vi "VGS Volume.vi"() -> ()   [LabVIEW 2022 SP3, in "LV_VGS.lvlib"]
uses:
  LV_VGS.lvlib
  typedefs/3D Size (I32).ctl
  RemoteControlClient/VGS_RemoteControlClient.lvclass
  Project/VGS_Project.lvclass
  VolumeDescriptor+File/VGS_VolumeDescriptor+File.lvclass
  VolumeDescriptor/VGS_VolumeDescriptor.lvclass
  ManufacturerInfo/VGS_ManufacturerInfo.lvclass
  ComponentInfo/VGS_ComponentInfo.lvclass
panel:
  out "Save Time, ms":u32
  # "Original Volume Example rewritten in LabVIEW"
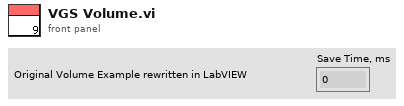
[diagram p1: front panel]
types:
  T1 = typedef "LV_VGS.lvlib/3D Size (I32).ctl" = cluster{"X":i32, "Y":i32, "Z":i32}
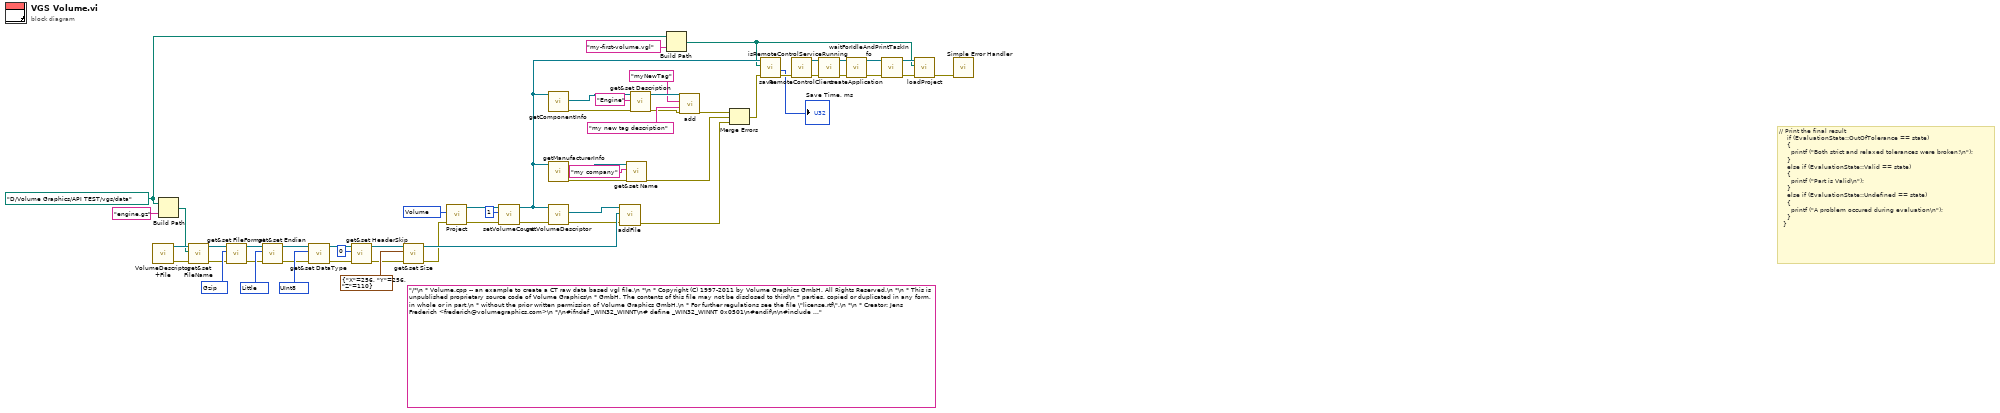
[diagram p0: block diagram]
diagram:
  w1 = 1448153088 items=["Volume"=1448153088, "Reconstruction"=1448153089] ("type")
  w46 = 1448157376 items=["UInt8"=1448157376, "Int8"=1448157377, "UInt16"=1448157378, "Int16"=1448157379, "UInt32"=1448157380, "Int32"=1448157381, "Float"=1448157382, "Rgb8"=1448157383] ("DataType")
  w49 = 1448157440 items=["Little"=1448157440, "Big"=1448157441] ("Endian")
  w52 = 1448157313 items=["Raw"=1448157312, "Gzip"=1448157313, "Tiff"=1448157314, "Jpeg"=1448157315, "Bmp"=1448157316, "Bir"=1448157317, "Toshiba"=1448157318, "Shimadzu"=1448157319, "Pnm"=1448157320, "Jpeg2"=1448157321, "Yxlon"=1448157322, "Hdf"=1448157323, "Dicom"=1448157324, "Imtec"=1448157325, "Aracor"=1448157326, "Fhg"=1448157327] ("FileFormat")
  w3 = path "D:/Volume Graphics/API TEST/vgs/data" ("replacementPattern")
  (unwired) "/*\n * Volume.cpp -- an example to create a CT raw data based vgl file.\n *\n * Copyright (C) 1997-2011 by Volume Graphics GmbH. All Rights Reserved.\n *\n * This is unpublished proprietary source code of Volume Graphics\n * GmbH. The contents of this file may not be disclosed to third\n * parties, copied or duplicated in any form, in whole or in part,\n * without the prior written permission of Volume Graphics GmbH.\n * For further regulations see the file \"license.rtf\".\n *\n * Creator: Jens Frederich <frederich@volumegraphics.com>\n */\n#ifndef _WIN32_WINNT\n# define _WIN32_WINNT 0x0501\n#endif\n\n#include <tchar.h>\n\n#include <vgs.project/project.h>\n\nusing namespace vgs::project;\nusing namespace vgs::project::volume;\n\nint _tmain (int argc, _TCHAR* argv[])\n{\n  Project* p = new Project (Project::Type::Volume);\n  assert (p != NULL);\n\n  // add single raw block file\n  {\n    VolumeDescriptor::File data;\n\n    data.setFileName   (\"D:/Volume Graphics/API TEST/vgs/data/engine.gz\");\n    data.setFileFormat (volume::FileFormat::Gzip);\n    data.setEndian     (volume::Endian::Little);\n    data.setDataType   (DataType::UInt8);\n    data.setHeaderSkip (0);\n    data.setSize       (Vector3<int> (256, 256, 110));\n    \n    p->setVolumeCount (1);\n    VolumeDescriptor* vd = p->getVolumeDescriptor (0);\n    assert (vd != NULL);\n\n    vd->addFile (data);\n  }\n\n  // add some meta data\n  {\n    ManufacturerInfo* mi = p->getManufacturerInfo ();\n    mi->setName (\"My company\");\n\n    ComponentInfo* ci = p->getComponentInfo ();\n    ci->setDescription (\"Engine\");\n\n    // add user defined tag\n    ci->add (\"myNewTag\", \"my new tag description\");\n\n    // add logo and preview\n    //p->setLogo    (\"c:/data/logo.png\");\n    //p->setPreview (\"c:/data/scene_preview.png\");\n  }\n\n  // create VG project\n  {\n    bool ok = true;\n\n    ok = p->save (std::string (\"D:/Volume Graphics/API TEST/vgs/data/my-first-volume1.vgl\"));\n    if (true != ok)\n    {\n      Error::ErrorCode err = Error::getLastError ();\n\t  printf(\"something is wrong, error code = %d\", err);\n      __debugbreak ();\n    }\n  }\n\n  // cleanup\n  if (p != NULL)\n  {\n    delete p;\n  }\n\n  return 0;\n}\n\n"
  # "// Print the final result\n    if (EvaluationState::OutOfTolerance == state)\n    {\n      printf (\"Both strict and relaxed tolerances were broken!\\n\");\n    }\n    else if (EvaluationState::Valid == state)\n    {\n      printf (\"Part is Valid\\n\");\n    }\n    else if (EvaluationState::Undefined == state)\n    {\n      printf (\"A problem occured during evaluation\\n\");\n    }\n  }"
  n1 = call "VolumeDescriptor+File.vi"() -> ("error out"=w54:errorcluster, "VGS_VolumeDescriptor+File out"=w57:refnum<class "VGS_VolumeDescriptor+File.lvclass">)  [unwired: 10 in]
  n2 = Build Path(base path=w3, name or relative path="engine.gz") -> (appended path=w55:path)
  n3 = call "get&set FileName.vi"("error in (no error)"=w54, "FileName"=w55, "VGS_VolumeDescriptor+File in"=w57) -> ("error out"=w51:errorcluster, "VGS_VolumeDescriptor+File out"=w53:refnum<class "VGS_VolumeDescriptor+File.lvclass">)  [unwired: 6 in, 1 out]
  n4 = call "get&set FileFormat.vi"("error in (no error)"=w51, "FileFormat"=w52, "VGS_VolumeDescriptor+File in"=w53) -> ("error out"=w48:errorcluster, "VGS_VolumeDescriptor+File out"=w50:refnum<class "VGS_VolumeDescriptor+File.lvclass">)  [unwired: 6 in, 1 out]
  n5 = call "get&set Endian.vi"("error in (no error)"=w48, "Endian"=w49, "VGS_VolumeDescriptor+File in"=w50) -> ("error out"=w45:errorcluster, "VGS_VolumeDescriptor+File out"=w47:refnum<class "VGS_VolumeDescriptor+File.lvclass">)  [unwired: 6 in, 1 out]
  n6 = call "get&set DataType.vi"("error in (no error)"=w45, "DataType"=w46, "VGS_VolumeDescriptor+File in"=w47) -> ("error out"=w42:errorcluster, "VGS_VolumeDescriptor+File out"=w44:refnum<class "VGS_VolumeDescriptor+File.lvclass">)  [unwired: 6 in, 1 out]
  n7 = call "get&set HeaderSkip.vi"("error in (no error)"=w42, "HeaderSkip"=0, "VGS_VolumeDescriptor+File in"=w44) -> ("error out"=w39:errorcluster, "VGS_VolumeDescriptor+File out"=w41:refnum<class "VGS_VolumeDescriptor+File.lvclass">)  [unwired: 6 in, 1 out]
  n8 = call "get&set Size.vi"("error in (no error)"=w39, "3D Size"=T1 {"X"=256, "Y"=256, "Z"=110}, "VGS_VolumeDescriptor+File in"=w41) -> ("error out"=w5:errorcluster, "VGS_VolumeDescriptor+File out"=w36:refnum<class "VGS_VolumeDescriptor+File.lvclass">)  [unwired: 6 in, 1 out]
  n9 = call "Project.vi"("error in (no error)"=w5, "type"=w1) -> ("error out"=w4:errorcluster, "VGS_Project out"=w38:refnum<class "VGS_Project.lvclass">)  [unwired: 8 in]
  n10 = call "setVolumeCount.vi"("error in (no error)"=w4, "VolumeCount"=u32 1, "VGS_Project in"=w38) -> ("error out"=w34:errorcluster, "VGS_Project out"=w24:refnum<class "VGS_Project.lvclass">)  [unwired: 7 in]
  n11 = call "getComponentInfo.vi"("VGS_Project in"=w24) -> ("error out"=w23:errorcluster, "VGS_ComponentInfo out"=w26:refnum<class "VGS_ComponentInfo.lvclass">)  [unwired: 8 in, 1 out]
  n12 = call "getManufacturerInfo.vi"("VGS_Project in"=w24) -> ("error out"=w21:errorcluster, "LV_VGS.lvlib:VGS_ManufacturerInfo.lvclass"=w25:refnum<class "VGS_ManufacturerInfo.lvclass">)  [unwired: 8 in, 1 out]
  n13 = call "getVolumeDescriptor.vi"("error in (no error)"=w34, "VGS_Project in"=w24) -> ("error out"=w33:errorcluster, "VGS_VolumeDescriptor out"=w35:refnum<class "VGS_VolumeDescriptor.lvclass">)  [unwired: 7 in, 1 out]
  n14 = call "addFile.vi"("error in (no error)"=w33, "LV_VGS.lvlib:VGS_VolumeDescriptor+File.lvclass"=w36, "VGS_VolumeDescriptor in"=w35) -> ("error out"=w18:errorcluster)  [unwired: 7 in, 1 out]
  n15 = call "get&set Name.vi"("error in (no error)"=w21, "Name"="my company", "VGS_ManufacturerInfo in"=w25) -> ("error out"=w20:errorcluster)  [unwired: 6 in, 2 out]
  n16 = call "get&set Description.vi"("error in (no error)"=w23, "Description"="Engine", "VGS_ComponentInfo in"=w26) -> ("error out"=w22:errorcluster, "VGS_ComponentInfo out"=w30:refnum<class "VGS_ComponentInfo.lvclass">)  [unwired: 6 in, 1 out]
  n17 = Build Path(base path=w3, name or relative path="my-first-volume.vgl") -> (appended path=w6:path)
  n18 = call "add.vi"("error in (no error)"=w22, "description"="my new tag description", "tag"="myNewTag", "VGS_ComponentInfo in"=w30) -> ("error out"=w19:errorcluster)  [unwired: 6 in, 1 out]
  n19 = Merge Errors(w19, w20, w18) -> (w17:errorcluster)
  n20 = call "save.vi"("error in (no error)"=w17, "Path"=w6, "VGS_Project in"=w24) -> ("error out"=w8:errorcluster, "Time, ms"=→"Save Time, ms":u32)  [unwired: 6 in, 1 out]
  n21 = call "RemoteControlClient.vi"("error in (no error)"=w8) -> ("error out"=w10:errorcluster, "VGS_RemoteControlClient out"=w9:refnum<class "VGS_RemoteControlClient.lvclass">)  [unwired: 9 in]
  n22 = call "isRemoteControlServiceRunning.vi"("error in (no error)"=w10, "VGS_RemoteControlClient in"=w9) -> ("error out"=w11:errorcluster, "VGS_RemoteControlClient out"=w12:refnum<class "VGS_RemoteControlClient.lvclass">)  [unwired: 7 in, 1 out]
  n23 = call "createApplication.vi"("error in (no error)"=w11, "VGS_RemoteControlClient in"=w12) -> ("error out"=w13:errorcluster, "VGS_RemoteControlClient out"=w16:refnum<class "VGS_RemoteControlClient.lvclass">)  [unwired: 8 in]
  n24 = call "waitForIdleAndPrintTaskInfo.vi"("error in (no error)"=w13, "VGS_RemoteControlClient in"=w16) -> ("error out"=w14:errorcluster, "VGS_RemoteControlClient out"=w15:refnum<class "VGS_RemoteControlClient.lvclass">)  [unwired: 8 in]
  n25 = call "loadProject.vi"("error in (no error)"=w14, "projectName"=w6, "VGS_RemoteControlClient in"=w15) -> ("error out"=w7:errorcluster)  [unwired: 7 in, 1 out]
  n26 = call <vilib>:"Simple Error Handler.vi"("error in (no error)"=w7) -> ()  [unwired: 4 in, 5 out]
